vi "NT Flush Data Updates.vi"(8 "error in (no error)":errorcluster) -> (0 "error out":errorcluster)   [LabVIEW 2020]
doc: "Flush any pending updates to connected Network Table and Smart Dashboard computers. Useful when you update a setpoint on a remote computer and want the robot to respond as quickly as possible.\n\nThis software is licensed. Open the labview\\readme\\WPI Robotics Library Open Source License.txt file for more information."
uses:
  ntcoreffi.dll
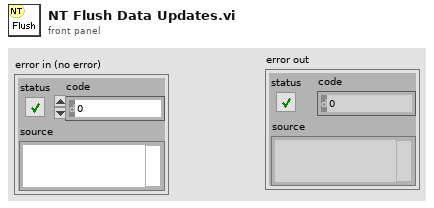
[diagram p1: front panel]
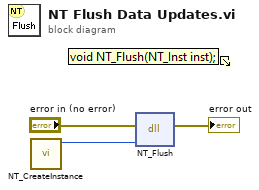
[diagram p0: block diagram]
diagram:
  n1 = call <vilib>:"NT_CreateInstance.vi"() -> ("InstanceHandle"=w1:u64)  [unwired: 10 in, 1 out]
  n2 = dll-call lib="ntcoreffi.*" fn="NT_Flush"(error in="error in (no error)", "InstHandle"=w1) -> (error out=→"error out":errorcluster)  [unwired: 4 in, 1 out]
